vi "configureTimer.vi"(8 "error in (no error)":errorcluster, 10 "channel":i32, 11 "K2602 in":refnum<class "K2602.lvclass">) -> (0 "error out":errorcluster, 3 "K2602 out":refnum<class "K2602.lvclass">)   [LabVIEW 2011, in "Hardware.lvlib" / "Channels.lvlib" / "K2602.lvclass"]
uses:
  K2602.lvclass
  K2602.lvclass/K2602.ctl
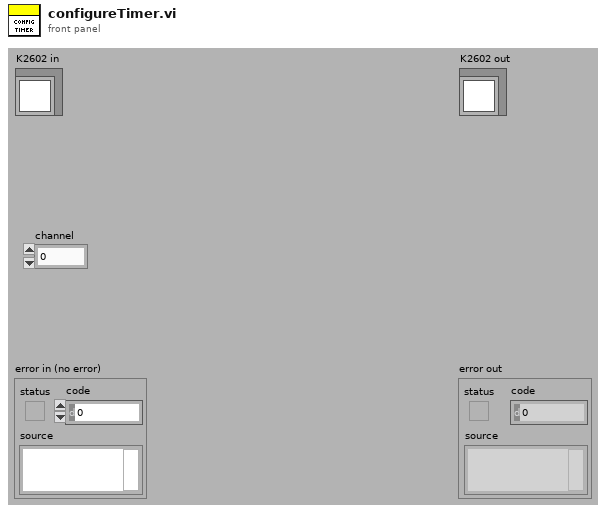
[diagram p1: front panel]
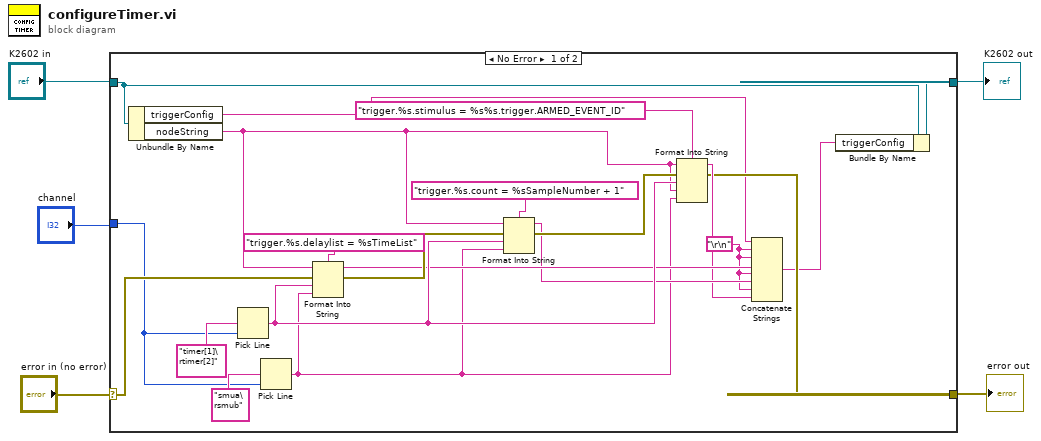
[diagram p0: block diagram]
diagram:
  n1 = case shown="No Error" "error in (no error)" {
    selector: "error in (no error)" -> [w25 w28]
    tunnel: [w14 w28] -> w3
    tunnel: [w12 w27] -> w4
    tunnel: "K2602 in" -> [w13 w27]
    tunnel: "channel" -> [w10 _]
    frame No Error {
      w9 = "\r\n"
      n2 = Unbundle By Name(w13) -> ("triggerConfig"=w8:string, "nodeString"=w7:string)
      n3 = Pick Line(multi-line string="timer[1]\rtimer[2]" ("options"), line index=w10) -> (output string=w19:string)  [unwired: 1 out]
      n4 = Pick Line(multi-line string="smua\rsmub" ("options"), line index=w10) -> (output string=w6:string)  [unwired: 1 out]
      n5 = Format Into String(format string="trigger.%s.delaylist = %sTimeList", initial string=w7, error in=w25, w19, w6) -> (resulting string=w17:string, error out=w22:errorcluster)
      n6 = Format Into String(format string="trigger.%s.count = %sSampleNumber + 1", initial string=w7, error in=w22, w19, w6) -> (resulting string=w16:string, error out=w20:errorcluster)
      n7 = Format Into String(format string="trigger.%s.stimulus = %s%s.trigger.ARMED_EVENT_ID", initial string=w7, error in=w20, w19, w7, w6) -> (resulting string=w15:string, error out=w14:errorcluster)
      n8 = Concatenate Strings(w8, w9, w9, w17, w9, w16, w9, w15) -> (w11:string)
      n9 = Bundle By Name(cluster=w13, "triggerConfig"=w11) -> (w12:refnum<class "K2602.lvclass">)
    }
    frame Error {
    }
  }
  "error out" <- w3
  "K2602 out" <- w4
